vi "ROS_Init_Topics.vi"() -> (0 "wl_out":T1={"topic port"=0, "Node"="", "topic"="", "type"="", "node port"=0, "error "={"status"=FALSE, "code"=0, "source"=""}, "Direction"=enum."Node", "Update (ms)"=1, "FIFO size"=1}, 1 "wr_out":T1={"topic port"=0, "Node"="", "topic"="", "type"="", "node port"=0, "error "={"status"=FALSE, "code"=0, "source"=""}, "Direction"=enum."Node", "Update (ms)"=1, "FIFO size"=1}, 2 "SP_W_out":T1={"topic port"=0, "Node"="", "topic"="", "type"="", "node port"=0, "error "={"status"=FALSE, "code"=0, "source"=""}, "Direction"=enum."Node", "Update (ms)"=1, "FIFO size"=1}, 3 "SP_V_out":T1={"topic port"=0, "Node"="", "topic"="", "type"="", "node port"=0, "error "={"status"=FALSE, "code"=0, "source"=""}, "Direction"=enum."Node", "Update (ms)"=1, "FIFO size"=1}, 4 "error out":errorcluster, 5 "scan_out":T1={"topic port"=0, "Node"="", "topic"="", "type"="", "node port"=0, "error "={"status"=FALSE, "code"=0, "source"=""}, "Direction"=enum."Node", "Update (ms)"=1, "FIFO size"=1})   [LabVIEW 2017]
doc: "Initialise ROS topics"
uses:
  <vilib>/Tufts CEEO ROS for LabVIEW Software/ROS/Code/SubVIs/_ROSControl.ctl
  <vilib>/Tufts CEEO ROS for LabVIEW Software/ROS/Code/SubVIs/_ROSDirection.ctl
  <vilib>/Tufts CEEO ROS for LabVIEW Software/ROS/Code/Console/Servers/ServerSubs/TopicDef.ctl
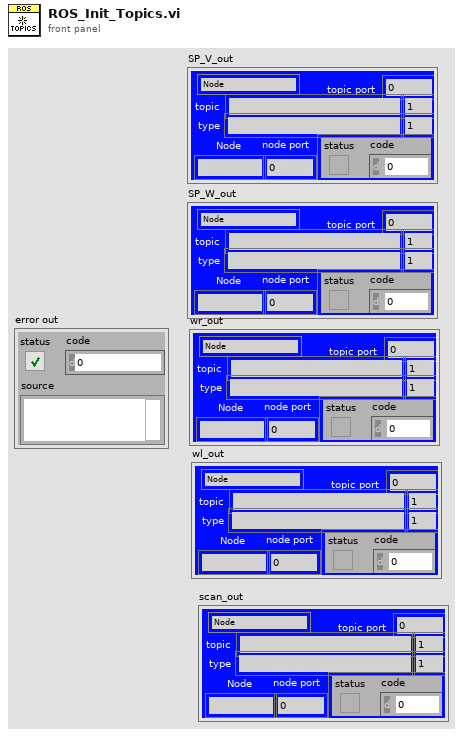
[diagram p1: front panel]
types:
  T1 = typedef "_ROSControl.ctl" = cluster{"topic port":u16, "Node":string, "topic":string, "type":string, "node port":u16, "error ":errorcluster, "Direction":T2, "Update (ms)":u16, "FIFO size":u16}
  T2 = typedef "_ROSDirection.ctl" = enum16{"Node", "Publisher", "Subscriber", "ServiceClient", "ServiceProvider"}
  T3 = typedef "TopicDef.ctl" = cluster{"Topic":string, "Type":string, "Action":T2, "Update (ms)":u16, "queue size":u16}
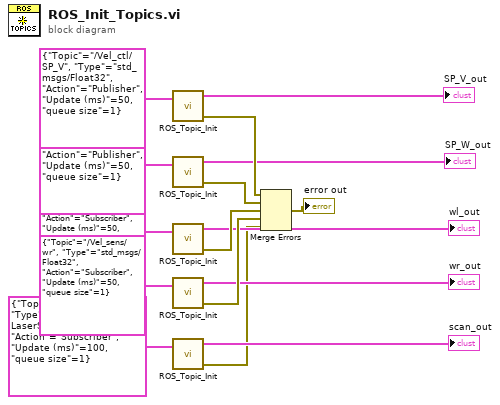
[diagram p0: block diagram]
diagram:
  n1 = call <vilib>:"ROS_Topic_Init.vi"("Definitions"=T3 {"Topic"="/Vel_ctl/SP_V", "Type"="std_msgs/Float32", "Action"=enum."Publisher", "Update (ms)"=50, "queue size"=1}) -> ("ROS out"=→"SP_V_out":T1, "error out"=w12:errorcluster)  [unwired: 2 in]
  n2 = call <vilib>:"ROS_Topic_Init.vi"("Definitions"=T3 {"Topic"="/Vel_ctl/SP_W", "Type"="std_msgs/Float32", "Action"=enum."Publisher", "Update (ms)"=50, "queue size"=1}) -> ("ROS out"=→"SP_W_out":T1, "error out"=w11:errorcluster)  [unwired: 2 in]
  n3 = call <vilib>:"ROS_Topic_Init.vi"("Definitions"=T3 {"Topic"="/Vel_sens/wl", "Type"="std_msgs/Float32", "Action"=enum."Subscriber", "Update (ms)"=50, "queue size"=1}) -> ("ROS out"=→"wl_out":T1, "error out"=w10:errorcluster)  [unwired: 2 in]
  n4 = call <vilib>:"ROS_Topic_Init.vi"("Definitions"=T3 {"Topic"="/Vel_sens/wr", "Type"="std_msgs/Float32", "Action"=enum."Subscriber", "Update (ms)"=50, "queue size"=1}) -> ("ROS out"=→"wr_out":T1, "error out"=w9:errorcluster)  [unwired: 2 in]
  n5 = call <vilib>:"ROS_Topic_Init.vi"("Definitions"=T3 {"Topic"="/scan", "Type"="sensor_msgs/LaserScan", "Action"=enum."Subscriber", "Update (ms)"=100, "queue size"=1}) -> ("ROS out"=→"scan_out":T1, "error out"=w1:errorcluster)  [unwired: 2 in]
  n6 = Merge Errors(w12, w11, w10, w9, w1) -> (→"error out":errorcluster)
